vi "Update Clock.vi"(6 "timeout (ms)":i32=5000, 8 "error in (no error)":errorcluster, 10 "Clock Update":T1, 11 "CIFCorePlugin in":refnum<class "CIFCorePlugin.lvclass">) -> (0 "error out":errorcluster, 3 "CIFCorePlugin out":refnum<class "CIFCorePlugin.lvclass">)   [LabVIEW 2021, in "CIFCorePlugin.lvclass"]
uses:
  CIFCorePlugin.lvclass
  CIFCorePlugin.lvclass/CIFCorePlugin.ctl
  CIFPluginManager/CIFPluginManager/gRPC/CIF_Manager_Client_Wrapper/CIFManagerClientWrapper.lvlib
  CIFUtilities/CIFClocks/Typedef/Timestamp Pair.ctl
  CIFUtilities/CIFClocks/CIFClocks.lvlib
  CIFUtilities/CIFClocks/Typedef/Clock Update.ctl
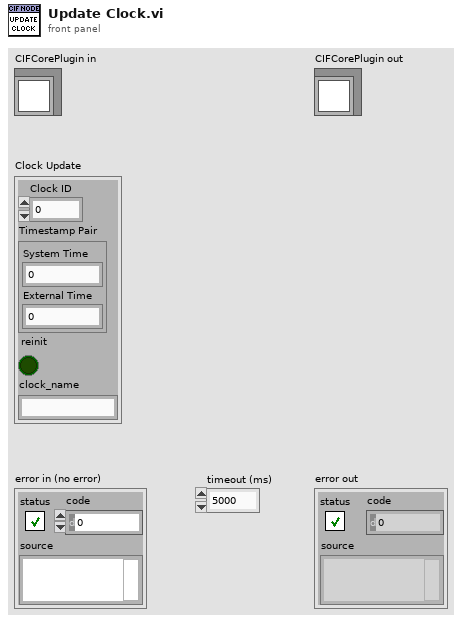
[diagram p1: front panel]
types:
  T1 = typedef "CIFClocks.lvlib/Clock Update.ctl" = cluster{"Clock ID":u8, "Timestamp Pair":T2, "reinit":bool, "clock_name":string}
  T2 = typedef "CIFClocks.lvlib/Timestamp Pair.ctl" = cluster{"System Time":i64, "External Time":i64}
  T3 = typedef "grpc-lvsupport-release.lvlib/grpcId.ctl" = u64
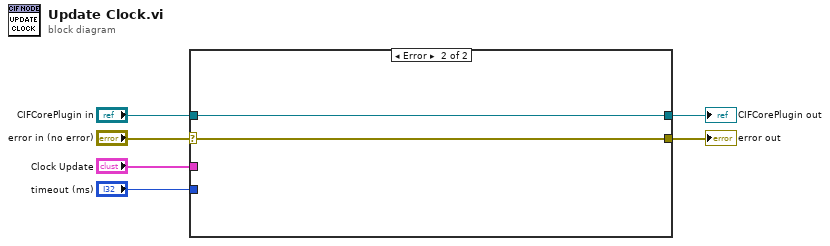
[diagram p0: block diagram]
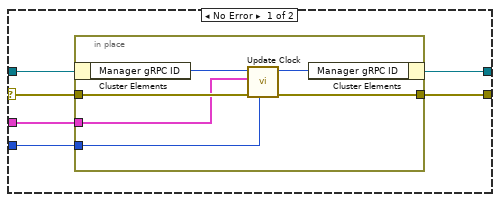
[diagram p2: hidden frame]
diagram:
  n1 = case shown="Error" "error in (no error)" {
    selector: "error in (no error)" -> [w12 w20]
    tunnel: [w11 w20] -> w5
    tunnel: [w10 w19] -> w3
    tunnel: "CIFCorePlugin in" -> [w9 w19]
    tunnel: "Clock Update" -> [w8 _]
    tunnel: "timeout (ms)" -> [w7 _]
    frame No Error {
      n2 = in-place {
        in-place-border: w12 -> [w18]
        in-place-border: [w17] -> w11
        in-place-border: w8 -> [w14]
        in-place-border: w7 -> [w13]
        n3 = in-place-cluster #1(w9) -> ("Manager gRPC ID"=w16:T3)
        n4 = call "Update Clock.vi"("timeout (ms)"=w13, "error in"=w18, "Clock Update"=w14, "gRPC ID in"=w16) -> ("error out"=w17:errorcluster, "gRPC ID out"=w15:T3)  [unwired: 6 in]
        n5 = in-place-cluster #1("Manager gRPC ID"=w15) -> (w10:refnum<class "CIFCorePlugin.lvclass">)
      }
    }
    frame Error {
    }
  }
  "error out" <- w5
  "CIFCorePlugin out" <- w3
